vi "Command Actuaute Cube.vi"(7 "Startup":bool) -> (2 "Actuate":bool, 4 "Reinit":bool, 6 "Completed":bool)   [LabVIEW 2017]
uses:
  Command Execution State.ctl
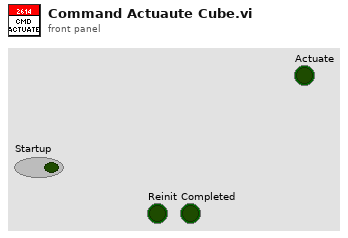
[diagram p1: front panel]
types:
  T1 = typedef "Command Execution State.ctl" = enum16{"Initialize", "Execute", "Finish"}
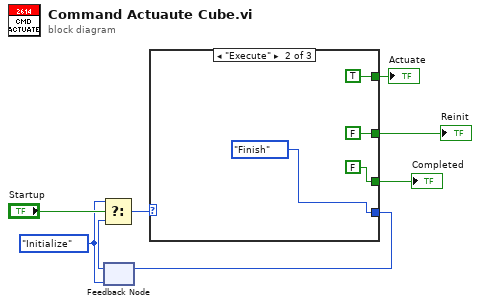
[diagram p0: block diagram]
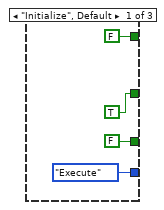
[diagram p2: hidden frame]
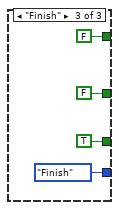
[diagram p3: hidden frame]
diagram:
  w6 = Command_Execution_State."Initialize" ("Play State")
  n1 = feedback #1(w6) -> (w5:T1)
  n2 = Select(t=w6, s="Startup", f=w5) -> (s? t:f=w7:T1)
  n3 = case shown="\"Execute\"" w7 {
    tunnel: [TRUE FALSE FALSE] -> w4
    tunnel: [FALSE TRUE FALSE] -> w1
    tunnel: [Command_Execution_State."Execute" ("Play State") Command_Execution_State."Finish" ("Play State") Command_Execution_State."Finish" ("Play State")] -> w3
    tunnel: [FALSE FALSE TRUE] -> w2
    frame "Initialize", Default {
    }
    frame "Execute" {
    }
    frame "Finish" {
    }
  }
  "Reinit" <- w4
  "Completed" <- w2
  "Actuate" <- w1
  n4 = feedback-in #1(w3) -> ()
